vi "get_positions_component.vi"(8 "error in (no error)":errorcluster, 10 "dimension (0/1/2 for x/y/z)":i32, 11 "PositionSignals in":refnum<class "PositionSignals.lvclass">) -> (0 "error out":errorcluster, 2 "x positions":sgl[](array[numeric]), 3 "PositionSignals out":refnum<class "PositionSignals.lvclass">)   [LabVIEW 2010, in "PositionSignals.lvclass"]
uses:
  PositionSignals.lvclass
  PositionSignals.lvclass/PositionSignals.ctl
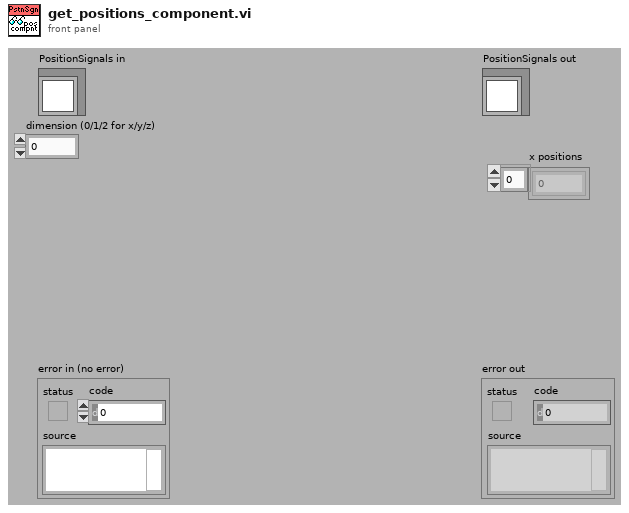
[diagram p1: front panel]
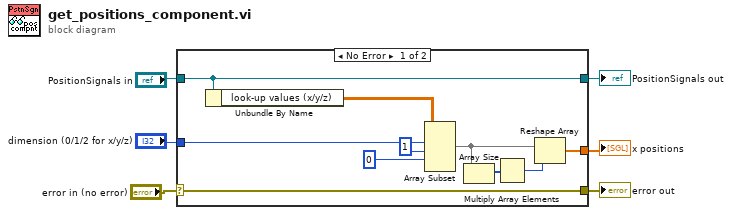
[diagram p0: block diagram]
diagram:
  n1 = case shown="No Error" "error in (no error)" {
    selector: "error in (no error)" -> [w16 w18]
    tunnel: [w16 w18] -> w5
    tunnel: [w15 w17] -> w3
    tunnel: "PositionSignals in" -> [w15 w17]
    tunnel: [w11 _] -> w2
    tunnel: "dimension (0/1/2 for x/y/z)" -> [w7 _]
    frame No Error {
      n2 = Unbundle By Name(w15) -> ("look-up values (x/y/z)"=w12:sgl[][])
      n3 = Array Subset(array=w12, index (row)=w7, length (row)=1 ("length"), index (col)=0 ("index")) -> (w10:sgl[][])  [unwired: 1 in]
      n4 = Array Size(array=w10) -> (size(s)=w8:i32[])
      n5 = Multiply Array Elements(1:w8) -> (0:w9:i32)
      n6 = Reshape Array(w10, w9) -> (w11:sgl[])
    }
    frame Error {
    }
  }
  "error out" <- w5
  "PositionSignals out" <- w3
  "x positions" <- w2
